vi "mainContainer.vi"() -> ()   [LabVIEW 2014]
panel:
  out "XY Graph":cluster{"Y":dbl[], "Y":dbl[]}[](graph)
  in  "B":bool
  in  "A":bool
  in  "G":bool
  in  "F":bool
  in  "E":bool
  in  "D":bool
  in  "C":bool
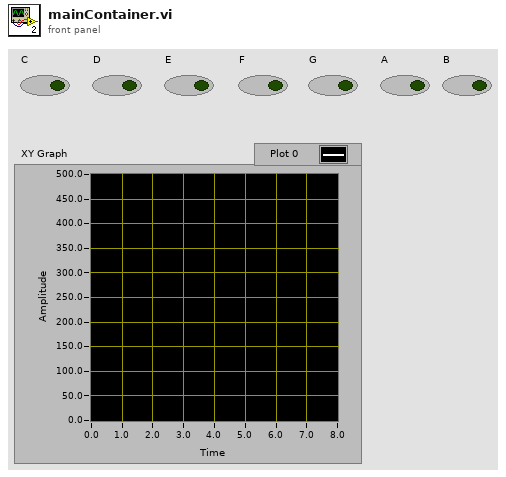
[diagram p1: front panel]
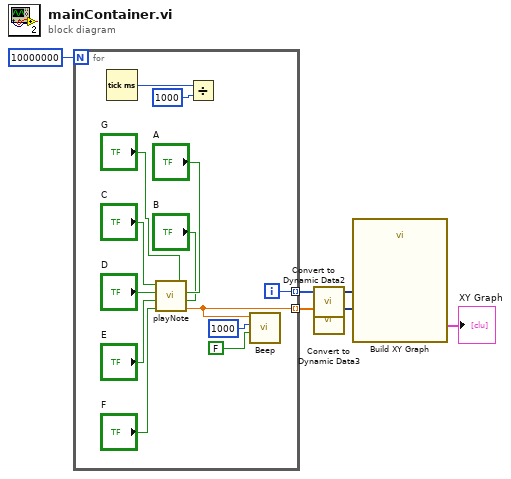
[diagram p0: block diagram]
diagram:
  n1 = for {
    N: 10000000 -> [_]
    tunnel: [w8] -> w2 mode=indexing
    tunnel: [w7] -> w3 mode=indexing
    i -> [w7]
    n2 = Tick Count (ms)() -> (millisecond timer value=w10:u32)
    n3 = call "playNote.vi"("B"="B", "A"="A", "G"="G", "F"="F", "E"="E", "D"="D", "C"="C") -> ("freq"=w8:dbl)
    n4 = Divide(x=w10, y=u32 1000) -> ()  [unwired: 1 out]
    n5 = call <vilib>:"Beep.vi"("use system alert? (T)"=FALSE, "duration (msec)"=u32 1000, "frequency (Hz)"=w8) -> ()  [unwired: 9 in]
  }
  n6 = call "Convert to Dynamic Data2"("Array"=w3) -> ("Dynamic Data Type"=w4:dynamicdata)  [unwired: 3 in]
  n7 = call "Convert to Dynamic Data3"("Array"=w2) -> ("Dynamic Data Type"=w1:dynamicdata)  [unwired: 3 in]
  n8 = call "Build XY Graph"("Y Input"=w1, "X Input"=w4) -> ("XY Graph"=→"XY Graph":cluster{"X":dbl[], "Y":dbl[]}[])  [unwired: 8 in, 1 out]
